vi "Set LED.vi"(8 "Error In":errorcluster, 10 "LED State":T1, 11 "Index":i32) -> (0 "Error Out":errorcluster)   [LabVIEW 2011, in "LVH-Interface-for-Kinect.lvlib"]
uses:
  <vilib>/LabVIEW Hacker/LVH-Interface-for-Kinect/LVH-Interface-for-Kinect.lvlib
  <vilib>/LabVIEW Hacker/LVH-Interface-for-Kinect/Public/Type Defs/LED State.ctl
  <vilib>/LabVIEW Hacker/LVH-Interface-for-Kinect/Public/lib/freenect_sync.dll
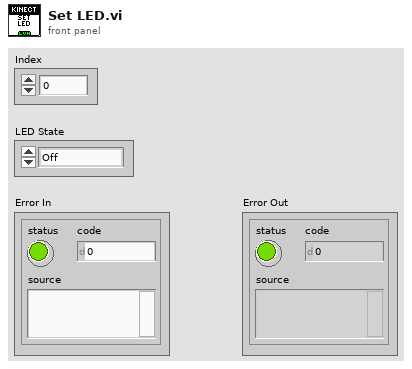
[diagram p1: front panel]
types:
  T1 = typedef "LVH-Interface-for-Kinect.lvlib/LED State.ctl" = enum16{"Off", "Green", "Red", "Yellow", "Blink Green", "Reserved", "Blink Red-Yellow"}
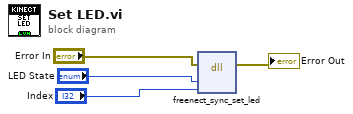
[diagram p0: block diagram]
diagram:
  n1 = dll-call lib="C:/Program Files (x86)/National Instruments/LabVIEW 2011/vi.lib/LabVIEW Hacker/LVH-Interface-for-Kinect/Public/lib/freenect_sync.dll" fn="freenect_sync_set_led"(error in="Error In", "LED State"="LED State", "Index"="Index") -> (error out=→"Error Out":errorcluster)  [unwired: 5 in, 1 out]
